vi "sprawdzenie zgodności ze wzorcem współrzędnych punktu.vi"(0 "Tekst":string, 1 "Wzór":string) -> (7 "Znaleziony tekst":string, 10 "Nieprawidłowy wzór":errorcluster)   [LabVIEW 2015, in "Biblioteka moduł map v3.lvlib" / "Konwersja wsp.lvlib" / "Obsługa błędów.lvlib"]
doc: "W polu \"tekst\" zostaje wprowadzony tekst będący współrzędnymi geograficznymi punktu. W ogólnym przypadku subVI nadaje się do dowolnego zastosowania w którym wprowadzamy jakiś tekst i wyszukujemy konkretnego wzorca. Jeżeli wzorzecz został odnaleziony zwracana jest prawda oraz w polu \"Znaleziony tekst\" zostaje wyświetlony tekst który jest zgodny ze wzorcem."
uses:
  <vilib>/regexp/Match Regular Expression.xnode
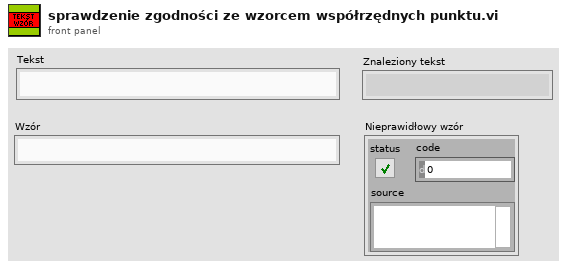
[diagram p1: front panel]
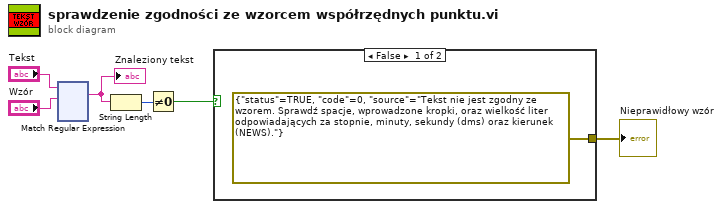
[diagram p0: block diagram]
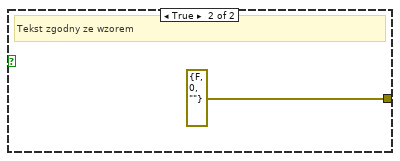
[diagram p2: hidden frame]
diagram:
  n1 = xnode "Match Regular Expression"("input string"="Tekst", "regular expression"="Wzór") -> ("whole match"=w2:string)  [unwired: 4 in, 4 out]
  "Znaleziony tekst" <- w2
  n2 = String Length(string=w2) -> (length=w5:i32)
  n3 = Not Equal To 0?(x=w5) -> (x != 0?=w1:bool)
  n4 = case shown="False" w1 {
    tunnel: [errorcluster {"status"=TRUE, "code"=0, "source"="Tekst nie jest zgodny ze wzorem. Sprawdź spacje, wprowadzone kropki, oraz wielkość liter odpowiadających za stopnie, minuty, sekundy (dms) oraz kierunek (NEWS)."} ("error constant") errorcluster {"status"=FALSE, "code"=0, "source"=""} ("error constant")] -> w3
    frame False {
    }
    frame True {
      # "Tekst zgodny ze wzorem"
    }
  }
  "Nieprawidłowy wzór" <- w3
